vi "Group Count.vi"(8 "error in (no error)":errorcluster, 11 "Framework Configuration in":refnum<class "Framework Configuration.lvclass">) -> (0 "error out":errorcluster, 2 "group count":i32, 3 "Framework Configuration out":refnum<class "Framework Configuration.lvclass">)   [LabVIEW 2019, in "DSF Core.lvlib" / "Framework Configuration.lvclass"]
uses:
  Framework Configuration.lvclass
  Framework Configuration.lvclass/Framework Configuration.ctl
  Plugin/Plugin Configuration.lvclass
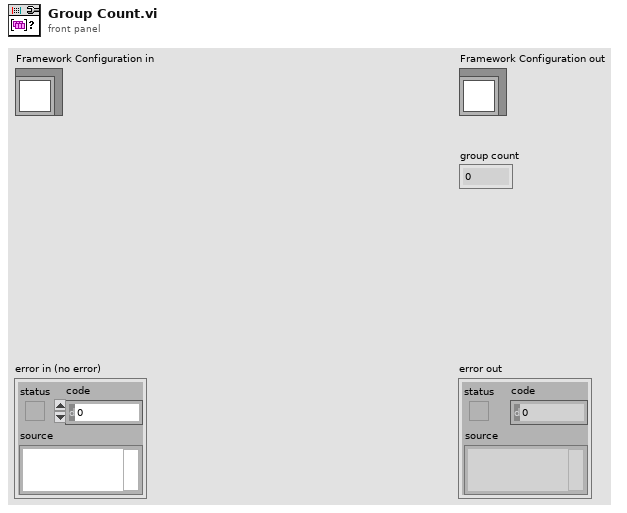
[diagram p1: front panel]
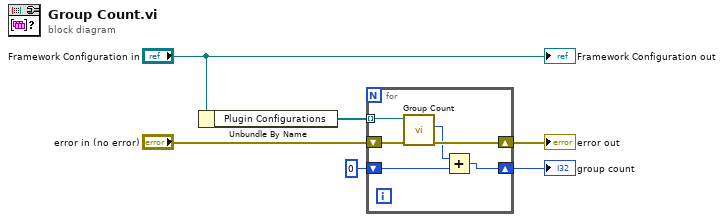
[diagram p0: block diagram]
diagram:
  n1 = Unbundle By Name("Framework Configuration in") -> ("Plugin Configurations"=w5:refnum<class "Plugin Configuration.lvclass">[])
  n2 = for {
    tunnel: w5 -> [w12] mode=indexing
    shift-right: [w11] -> w3
    shift-left: "error in (no error)" -> [w10]
    shift-right: [w8] -> w1
    shift-left: 0 -> [w7]
    n3 = call-dynamic "Group Count.vi"("error in (no error)"=w10, "Plugin Configuration in"=w12) -> ("error out"=w11:errorcluster, "group count"=w9:i32)  [unwired: 7 in, 1 out]
    n4 = Add(x=w9, y=w7) -> (x+y=w8:i32)
  }
  "error out" <- w3
  "group count" <- w1
  "Framework Configuration out" <- "Framework Configuration in"
